vi "Temperature Limit.vi"() -> ()   [LabVIEW 2015]
doc: "This VI simulates the acquisition of temperature, graphs the temperature, and notifies the user if the temperature is over the limit."
panel:
  in  "Start":bool
  in  "Delta t (ms)":i32(slide)=400 scale=50.0..500.0
  in  "Stop":bool
  in  "High Limit":dbl=28.0 format="%.2f"
  out "Temperature":cluster{"Temperature":dbl, "High Limit":dbl}(graph)={"Temperature"=85.88749999999999, "High Limit"=80.0}
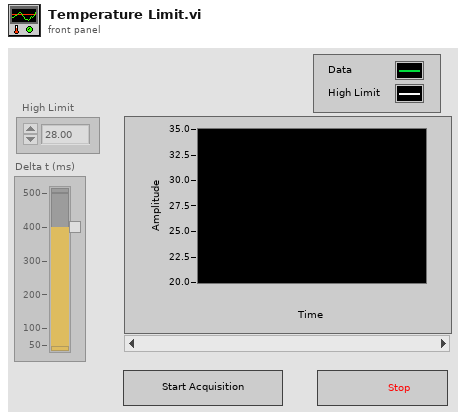
[diagram p1: front panel]
types:
  T1 = enum8{"Enabled", "Disabled", "Disabled and Grayed Out"}
  T2 = cluster{"Temperature Value":dbl, "High Limit":dbl}
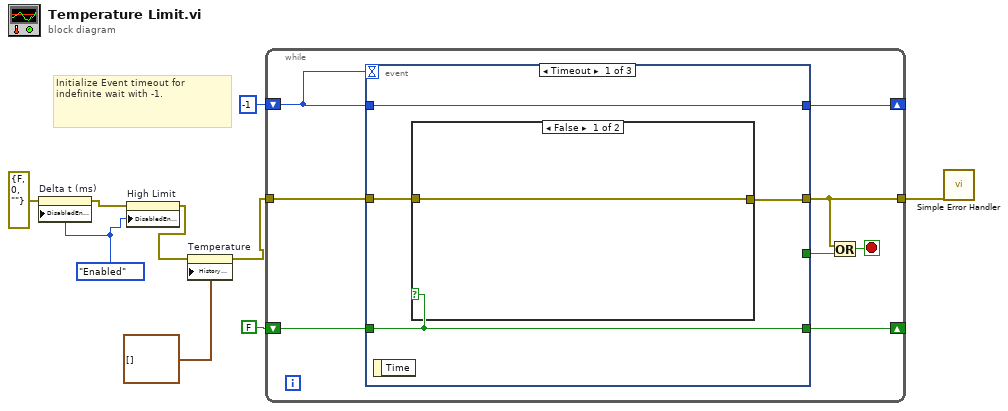
[diagram p0: block diagram]
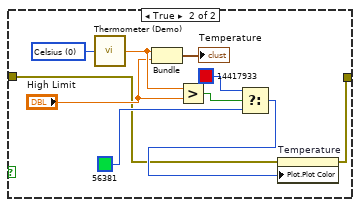
[diagram p2: hidden frame]
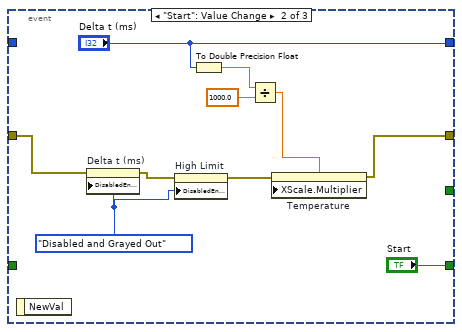
[diagram p3: hidden frame]
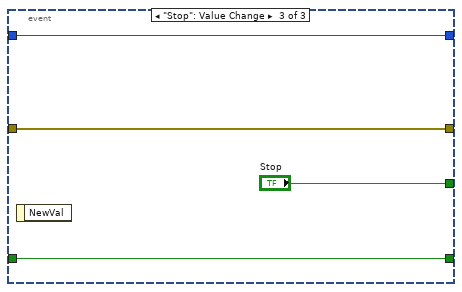
[diagram p4: hidden frame]
diagram:
  w6 = T1."Enabled" ("Disabled")
  # "Initialize Event timeout for indefinite wait with -1."
  n1 = property on="Delta t (ms)" class="Slide (strict)"(error in=errorcluster {"status"=FALSE, "code"=0, "source"=""} ("error in (no error)"), "DisabledEnum"=w6) -> (error out=w5:errorcluster)  [unwired: 1 in, 1 out]
  n2 = property on="High Limit" class="DigNum (strict)"(error in=w5, "DisabledEnum"=w6) -> (error out=w3:errorcluster)  [unwired: 1 in, 1 out]
  n3 = property on="Temperature" class="WFChart (strict)"(error in=w3, "History Data"=cluster{"Temperature":dbl, "High Limit":dbl}[] []) -> (error out=w2:errorcluster)  [unwired: 1 in, 1 out]
  n4 = while {
    tunnel: w2 -> [w17]
    tunnel: [w15] -> w8
    shift-right: [w13] -> _
    shift-left: FALSE ("Start") -> [w12]
    shift-right: [w11] -> _
    shift-left: -1 ("Delta t (ms)") -> [w10]
    stop <- w16 stop-if-true
    n5 = event shown="[0] Timeout" {
      selector: _ -> [_ _ _]
      dyn-events: _ -> [_ _ _]
      timeout: w10 -> [_ _ _]
      tunnel: [_ _ "Stop"] -> w14
      tunnel: w17 -> [w19 w41 w45]
      tunnel: [w18 w38 w45] -> w15
      tunnel: [w20 "Start" w44] -> w13
      tunnel: w12 -> [w20 _ w44]
      tunnel: [w21 "Delta t (ms)" w43] -> w11
      tunnel: w10 -> [w21 _ w43]
      event Timeout {
        n6 = event-data() -> ()  [unwired: 1 in, 1 out]
        n7 = case shown="False" w20 {
          tunnel: w19 -> [w22 w24]
          tunnel: [w22 w23] -> w18
          frame False {
          }
          frame True {
            w31 = u16 0 items=["Celsius", "Fahrenheit"] ("Units (0: Celsius)")
            n8 = call "Thermometer (Demo).vi"("Units (0: Celsius)"=w31) -> ("Temperature Value"=w30:dbl)
            n9 = Bundle("Temperature Value"=w30, "High Limit"="High Limit") -> (→"Temperature":T2)  [unwired: 1 in]
            n10 = Greater?(x=w30, y="High Limit") -> (0:w28:bool)
            n11 = Select(t=u32 14417933, s=w28, f=u32 56381) -> (s? t:f=w26:u32)
            n12 = property on="Temperature" class="WFChart (strict)"(error in=w24, "Plot.Plot Color"=w26) -> (error out=w23:errorcluster)  [unwired: 1 in, 1 out]
          }
        }
      }
      event "Start": Value Change {
        w37 = T1."Disabled and Grayed Out" ("Disabled")
        n13 = event-data() -> ()  [unwired: 1 in, 1 out]
        n14 = property on="Delta t (ms)" class="Slide (strict)"(error in=w41, "DisabledEnum"=w37) -> (error out=w40:errorcluster)  [unwired: 1 in, 1 out]
        n15 = property on="High Limit" class="DigNum (strict)"(error in=w40, "DisabledEnum"=w37) -> (error out=w39:errorcluster)  [unwired: 1 in, 1 out]
        n16 = To Double Precision Float(number="Delta t (ms)") -> (double precision float=w35:dbl)
        n17 = Divide(x=w35, y=1000.0) -> (x/y=w34:dbl)
        n18 = property on="Temperature" class="WFChart (strict)"(error in=w39, "XScale.Multiplier"=w34) -> (error out=w38:errorcluster)  [unwired: 1 in, 1 out]
      }
      event "Stop": Value Change {
        n19 = event-data() -> ()  [unwired: 1 in, 1 out]
      }
    }
    n20 = Or(x=w15, y=w14) -> (x .or. y?=w16:bool)
  }
  n21 = call <vilib>:"Simple Error Handler.vi"("error in (no error)"=w8) -> ()  [unwired: 4 in, 5 out]
